vi "Set Meta Data (TCP Clst).vi"(7 "meta data":T2[](array[typedef]), 8 "error in":errorcluster, 11 "connection info in":T1) -> (0 "error out":errorcluster, 3 "connection info out":T1)   [LabVIEW 2010, in "NI STM.lvlib"]
doc: "Assigns the meta data cluster associated with this STM session."
uses:
  NI STM.lvlib
  TCP Connection Info.ctl
  SubVIs/MetaDataElement.ctl
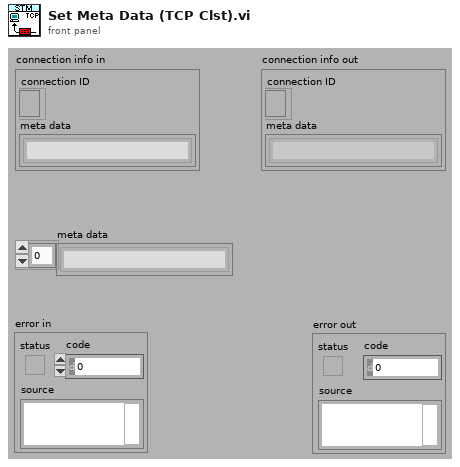
[diagram p1: front panel]
types:
  T1 = typedef "NI STM.lvlib/TCP Connection Info.ctl" = cluster{"connection ID":refnum<k5>, "meta data":T2[]}
  T2 = typedef "NI STM.lvlib/MetaDataElement.ctl" = string
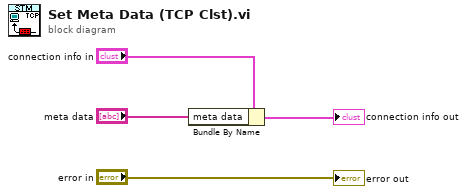
[diagram p0: block diagram]
diagram:
  n1 = Bundle By Name(cluster="connection info in", "meta data"="meta data") -> (→"connection info out":T1)
  "error out" <- "error in"
